vi "Default Format.vi"(10 "MultiErrors":T1[](array[typedef]), 11 "Max Errors":bool) -> (2 "error":errorcluster)   [LabVIEW 2020, in "VolatusErrorUtilities.lvlib" / "MultiError Formatter.lvclass"]
uses:
  MultiError Formatter.lvclass
  MultiError.ctl
  VolatusErrorUtilities.lvlib
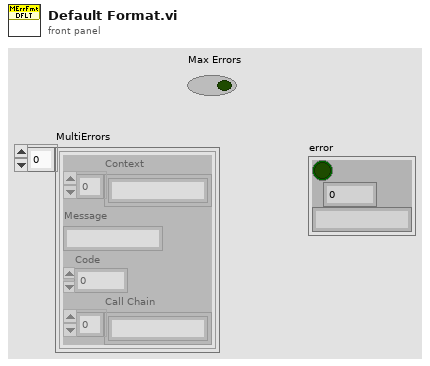
[diagram p1: front panel]
types:
  T1 = typedef "VolatusErrorUtilities.lvlib/MultiError.ctl" = cluster{"Context":string[], "Message":string, "Code":i32, "Call Chain":string[]}
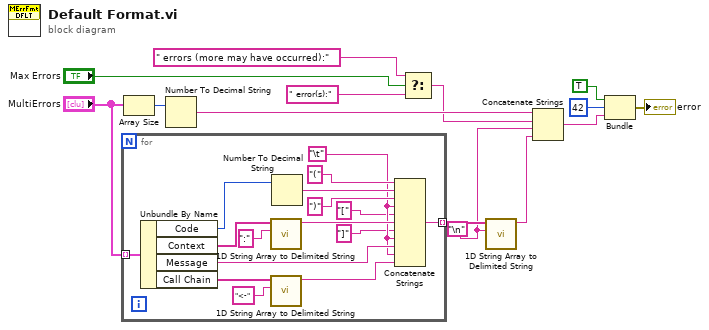
[diagram p0: block diagram]
diagram:
  w7 = "\n"
  n1 = for {
    tunnel: "MultiErrors" -> [w30] mode=indexing
    tunnel: [w17] -> w10 mode=indexing
    w19 = "\t"
    n2 = Unbundle By Name(w30) -> ("Code"=w25:i32, "Context"=w27:string[], "Message"=w20:string, "Call Chain"=w29:string[])
    n3 = call <vilib>:"1D String Array to Delimited String.vi"("delimiter"=":", "string array"=w27) -> ("delimited string"=w21:string)  [unwired: 9 in]
    n4 = call <vilib>:"1D String Array to Delimited String.vi"("delimiter"="<-", "string array"=w29) -> ("delimited string"=w18:string)  [unwired: 9 in]
    n5 = Number To Decimal String(number=w25) -> (decimal integer string=w24:string)  [unwired: 1 in]
    n6 = Concatenate Strings("(" ("string"), w24, ")" ("string"), w19, "[" ("string"), w21, "]" ("string"), w19, w20, w19, w18) -> (w17:string)
  }
  n7 = Array Size(array="MultiErrors") -> (size(s)=w9:i32)
  n8 = Number To Decimal String(number=w9) -> (decimal integer string=w8:string)  [unwired: 1 in]
  n9 = Select(t=" errors (more may have occurred):", s="Max Errors", f=" error(s):" ("string")) -> (s? t:f=w2:string)
  n10 = call <vilib>:"1D String Array to Delimited String.vi"("delimiter"=w7, "string array"=w10) -> ("delimited string"=w6:string)  [unwired: 9 in]
  n11 = Concatenate Strings(w8, w2, w7, w6) -> (w11:string)
  n12 = Bundle(TRUE, 42, w11) -> (→"error":errorcluster)  [unwired: 1 in]
